vi "Parse Menu Tag.vi"(11 "Tag":string) -> (1 "String":string, 2 "Int":i32, 3 "Menu Tag":T1)   [LabVIEW 2022 SP3, in "FlexBlocks Support.lvlib"]
uses:
  FlexBlocks Support.lvlib
  Menu Tag.ctl
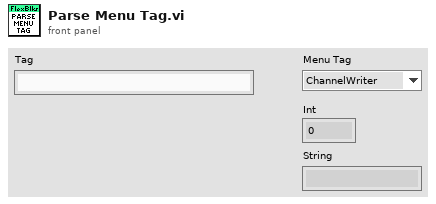
[diagram p1: front panel]
types:
  T1 = typedef "FlexBlocks Support.lvlib/Menu Tag.ctl" = enum16{"ChannelWriter", "LossyReader", "LosslessReader", "EventReader", "SmolMode"}
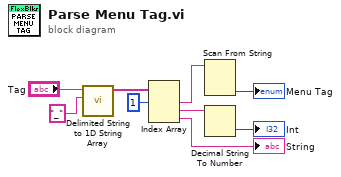
[diagram p0: block diagram]
diagram:
  n1 = call <vilib>:"Delimited String to 1D String Array.vi"("delimiter"="_", "delimited string"="Tag") -> ("string array"=w7:string[])  [unwired: 9 in]
  n2 = Index Array(array=w7, index #1=1 ("index")) -> (element #1=w5:string, element #2=w3:string, element #3=→"String":string)  [unwired: 2 in]
  n3 = Scan From String(input string=w5) -> (output 1=→"Menu Tag":T1)  [unwired: 4 in, 3 out]
  n4 = Decimal String To Number(string=w3) -> (number=→"Int":i32)  [unwired: 2 in, 1 out]
